vi "MoveSingleAxis.vi"(8 "Set velocity?":bool=TRUE, 9 "Velocity":sgl, 10 "Position":sgl, 11 "Axis info":T1={"System #"=0, "Axis ID"="", "Multiplier"=1.0}) -> ()   [LabVIEW 2011]
uses:
  PI_Axis.ctl
  PIAxisInfoGlobal.vi
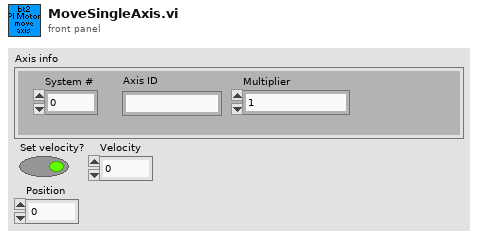
[diagram p1: front panel]
types:
  T1 = typedef "PI_Axis.ctl" = cluster{"System #":i32, "Axis ID":string, "Multiplier":dbl}
  T2 = typedef "GCS_Interface.ctl" = cluster{"MOV":refnum<vi>, "VEL":refnum<vi>, "VEL?":refnum<vi>, "POS?":refnum<vi>, "TMX?":refnum<vi>, "#7 (Ready?)":refnum<vi>, "FPL":refnum<vi>, "FNL":refnum<vi>}
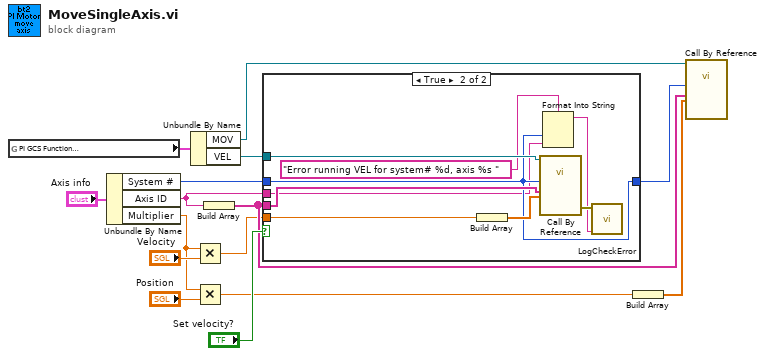
[diagram p0: block diagram]
diagram:
  n1 = global read "PIAxisInfoGlobal.vi" "PI GCS Function\nReferences"() -> (w15:T2)
  n2 = Unbundle By Name("Axis info") -> ("System #"=w5:i32, "Axis ID"=w1:string, "Multiplier"=w9:dbl)
  n3 = Unbundle By Name(w15) -> ("MOV"=w14:refnum<vi>, "VEL"=w6:refnum<vi>)
  n4 = Multiply(x=w9, y="Velocity") -> (x*y=w3:dbl)
  n5 = Multiply(x=w9, y="Position") -> (x*y=w8:dbl)
  n6 = Build Array(w1) -> (w4:string[])
  n7 = case shown="True" "Set velocity?" {
    tunnel: w6 -> [_ w25]
    tunnel: w5 -> [w16 w19]
    tunnel: w4 -> [_ w24]
    tunnel: w3 -> [_ w23]
    tunnel: [w16 w19] -> w2
    tunnel: w1 -> [_ w18]
    frame False {
    }
    frame True {
      n8 = Build Array(w23) -> (w22:dbl[])
      n9 = call-by-ref "?"(reference=w25, "System no."=w19, "Axes to set"=w24, "Velocity values"=w22) -> ("error out"=w21:errorcluster)  [unwired: 16 in, 3 out]
      n10 = Format Into String(format string="Error running VEL for system# %d, axis %s " ("Msg"), w19, w18) -> (resulting string=w17:string)  [unwired: 2 in, 1 out]
      n11 = call "LogCheckError.vi"("Msg"=w17, "error in (no error)"=w21) -> ()  [unwired: 10 in]
    }
  }
  n12 = Build Array(w8) -> (w7:dbl[])
  n13 = call-by-ref "?"(reference=w14, "System no."=w2, "Axes to move"=w4, "Position values"=w7) -> ()  [unwired: 17 in, 3 out]
